vi "Test Basic Deployment.vi"(8 "error in (no error)":errorcluster, 11 "Scalar Channels Testing in":refnum<class "Scalar Channels Testing.lvclass">) -> (0 "error out":errorcluster, 2 "System Definition Information":T1, 3 "Scalar Channels Testing out":refnum<class "Scalar Channels Testing.lvclass">)   [LabVIEW 2019, in "Scalar Channels Testing.lvclass"]
uses:
  Scalar Channels Testing.lvclass
  C:/Program Files (x86)/National Instruments/LabVIEW 2019/vi.lib/NI/NI VeriStand Development Tools/NI Veristand Test Utilities/VeriStandTestCase/VeriStandTestCase.lvclass
  <vilib>/NI/NI VeriStand Development Tools/NI Veristand Test Utilities/VeriStandTestUtilities/SystemDefinitionInformation.ctl
  <vilib>/NI/NI VeriStand Development Tools/NI Veristand Test Utilities/VeriStandTestUtilities/TargetInformation.ctl
  <vilib>/NI/NI VeriStand Development Tools/NI Veristand Test Utilities/VeriStandTestUtilities/ChassisInformation.ctl
  <vilib>/NI/NI VeriStand Development Tools/NI Veristand Test Utilities/VeriStandTestUtilities/VeriStandTestUtilities.lvlib
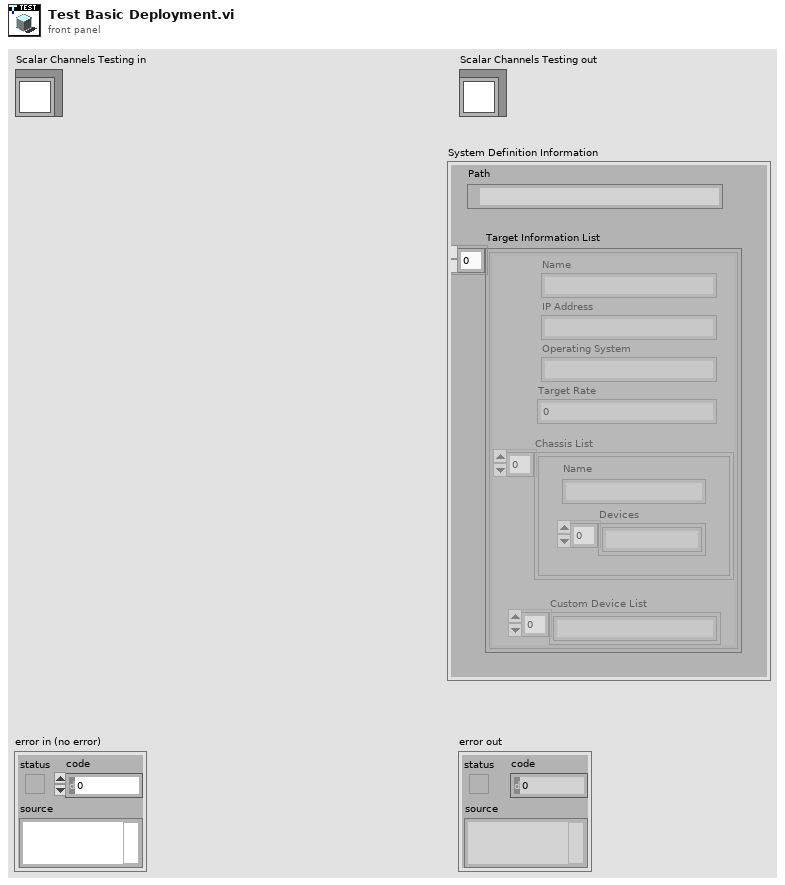
[diagram p1: front panel]
types:
  T1 = typedef "VeriStandTestUtilities.lvlib/SystemDefinitionInformation.ctl" = cluster{"Path":path, "Target Information List":T2[]}
  T2 = typedef "VeriStandTestUtilities.lvlib/TargetInformation.ctl" = cluster{"Name":string, "IP Address":string, "Operating System":string, "Target Rate":dbl, "Chassis List":T3[], "Custom Device List":string[]}
  T3 = typedef "VeriStandTestUtilities.lvlib/ChassisInformation.ctl" = cluster{"Name":string, "Devices":string[]}
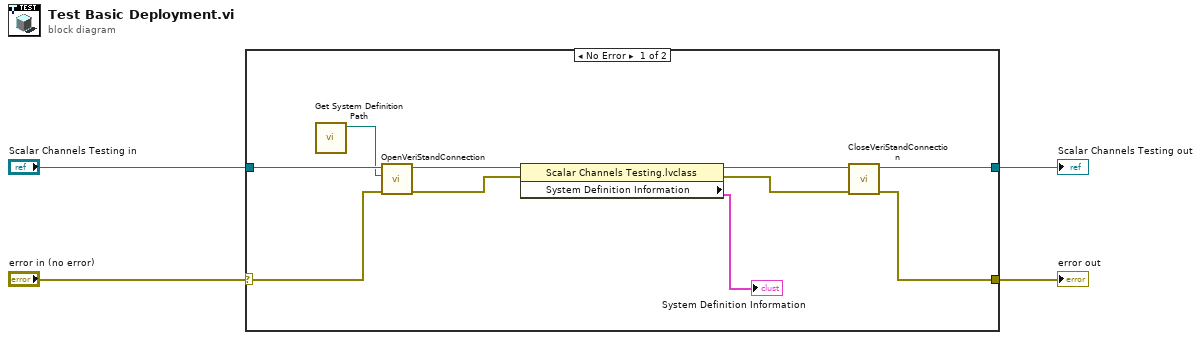
[diagram p0: block diagram]
diagram:
  n1 = case shown="No Error" "error in (no error)" {
    selector: "error in (no error)" -> [w7 w16]
    tunnel: [w6 w16] -> w3
    tunnel: [w8 w15] -> w1
    tunnel: "Scalar Channels Testing in" -> [w9 w15]
    frame No Error {
      n2 = call "Get System Definition Path.vi"() -> ("System Definition path"=w5:path)  [unwired: 11 in]
      n3 = call-dynamic "OpenVeriStandConnection.vi"("error in (no error)"=w7, "System Definition File"=w5, "VeriStand Test Case in"=w9) -> ("error out"=w13:errorcluster, "VeriStand Test Case out"=w14:refnum<class "Scalar Channels Testing.lvclass">)  [unwired: 6 in, 1 out]
      n4 = property class="Scalar Channels Testing.lvclass"(reference=w14, error in=w13) -> (reference out=w12:refnum<class "Scalar Channels Testing.lvclass">, error out=w10:errorcluster, "System Definition Information"=→"System Definition Information":T1)
      n5 = call-dynamic "CloseVeriStandConnection.vi"("error in (no error)"=w10, "VeriStand Test Case in"=w12) -> ("error out"=w6:errorcluster, "VeriStand Test Case out"=w8:refnum<class "Scalar Channels Testing.lvclass">)  [unwired: 8 in]
    }
    frame Error {
    }
  }
  "error out" <- w3
  "Scalar Channels Testing out" <- w1
